vi "New Abstract Group.vi"(8 "error in (no error)":errorcluster, 10 "Group Config":refnum<class "Group Config.lvclass">, 11 "ChannelService in":refnum<class "ChannelService.lvclass">) -> (0 "error out":errorcluster, 2 "Group":refnum<class "GroupAbstract.lvclass">, 3 "ChannelService out":refnum<class "ChannelService.lvclass">)   [LabVIEW 2020, in "Vecto.lvlib" / "ChannelService.lvclass"]
uses:
  ChannelService.lvclass
  ChannelService.lvclass/ChannelService.ctl
  GroupAbstract/GroupAbstract.lvclass
  Group Config/Group Config.lvclass
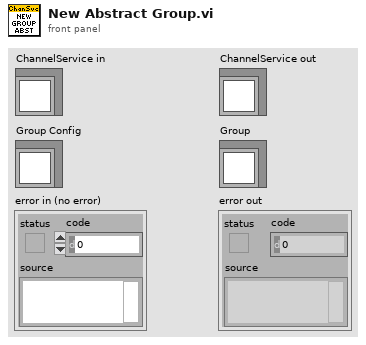
[diagram p1: front panel]
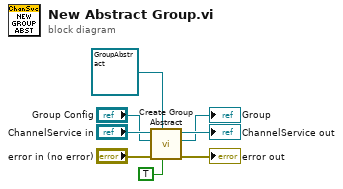
[diagram p0: block diagram]
diagram:
  n1 = call "Create Group Abstract.vi"("Skip Type Check (F)"=TRUE, "Group Type"=refnum<class "GroupAbstract.lvclass"> refnum ("Vecto.lvlib:GroupAbstract.lvclass"), "error in (no error)"="error in (no error)", "Group Config"="Group Config", "ChannelService in"="ChannelService in") -> ("error out"=→"error out":errorcluster, "Group"=→"Group":refnum<class "GroupAbstract.lvclass">, "ChannelService out"=→"ChannelService out":refnum<class "ChannelService.lvclass">)  [unwired: 4 in]
